vi "Create.vi"(8 "error in (no error)":errorcluster, 10 "Callbacks Only? (False)":bool, 11 "Mode (Buffered)":T1=enum."Message") -> (0 "error out":errorcluster, 3 "Websocket Server out":refnum<class "Websocket Server.lvclass">)   [LabVIEW 2020, in "Stream-Websocket.lvlib" / "Websocket Server.lvclass"]
uses:
  Websocket Server.lvclass
  Websocket Server.lvclass/Websocket Server.ctl
  <vilib>/IlluminatedG/lv-stream/stream/Mode.ctl
  <vilib>/IlluminatedG/lv-stream/Stream.lvlib
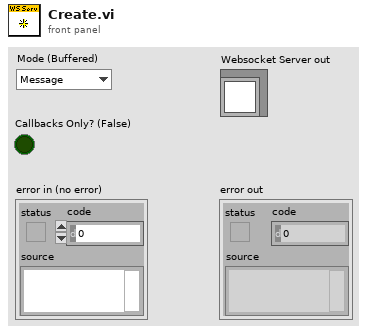
[diagram p1: front panel]
types:
  T1 = typedef "Stream.lvlib/Mode.ctl" = enum16{"Raw", "Buffered", "LineTerm", "Message"}
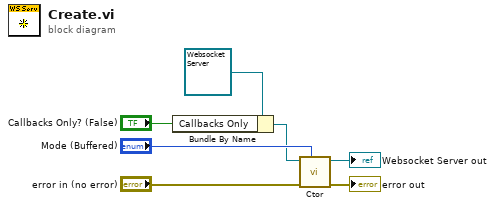
[diagram p0: block diagram]
diagram:
  n1 = Bundle By Name(cluster=refnum<class "Websocket Server.lvclass"> refnum ("Websocket Server in"), "Callbacks Only"="Callbacks Only? (False)") -> (w2:refnum<class "Websocket Server.lvclass">)
  n2 = call-dynamic "Ctor.vi"("Mode (Raw)"="Mode (Buffered)", "error in (no error)"="error in (no error)", "Websocket Server in"=w2) -> ("error out"=→"error out":errorcluster, "Websocket Server out"=→"Websocket Server out":refnum<class "Websocket Server.lvclass">)  [unwired: 7 in]
